vi "Get Zoom Parameter.vi"(8 "error in (no error)":errorcluster, 11 "Stream":refnum<data-value>) -> (0 "error out":errorcluster, 2 "Value":i32, 3 "Stream (duplicate)":refnum<data-value>)   [LabVIEW 2020, in "g_ar_toolkit.capture.lvlib" / "CameraStream.lvclass"]
uses:
  CameraStream.lvclass
  Camera Parameters.ctl
  CameraStream.lvclass/CameraStream.ctl
  <vilib>/Utility/error.llb/Error Cluster From Error Code.vi
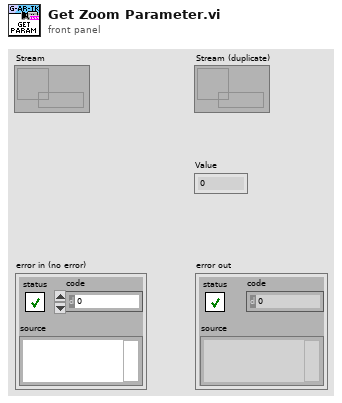
[diagram p1: front panel]
types:
  T1 = typedef "g_ar_toolkit.capture.lvlib/CameraStream.lvclass/Camera Parameters.ctl" = enum8{"EXPOSURE", "FOCUS", "ZOOM", "GAIN", "WHITE_BALANCE_TEMPERATURE", "BRIGHTNESS", "CONTRAST", "SATURATION", "GAMMA", "HUE", "SHARPNESS", "BACKLIGHT_COMPENSATION", "POWER_LINE_FREQUENCY"}
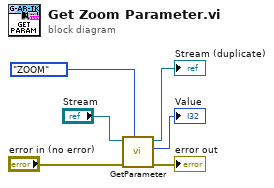
[diagram p0: block diagram]
diagram:
  n1 = call "GetParameter.vi"("Camera Parameter"=Camera_Parameters."ZOOM", "error in (no error)"="error in (no error)", "Stream"="Stream") -> ("error out"=→"error out":errorcluster, "Value"=→"Value":i32, "Stream (duplicate)"=→"Stream (duplicate)":refnum<data-value>)  [unwired: 6 in]
